vi "roboRIO v1.0 Reserve Encoder.vi"(7 "Allow multiple opens?":bool, 8 "error in (no error)":errorcluster, 10 "Encoder Channel":T2, 11 "myRIO FPGA Ref Out":T1) -> (0 "error out":errorcluster)   [LabVIEW 2021]
uses:
  <vilib>/myRIO/Common/Instrument Driver Framework/myRIO v1.0/Encoder/typedefs/Encoder Channels Enum.ctl
  <vilib>/myRIO/Common/Instrument Driver Framework/Utilities/typedefs/Generic FPGA Reference.ctl
  <vilib>/myRIO/Common/Instrument Driver Framework/roboRIO v1.0/Resource Manager/vis/roboRIO v1.0 Create Configuration List.vi
  <vilib>/myRIO/Common/Instrument Driver Framework/roboRIO v1.0/Resource Manager/vis/roboRIO v1.0 Reserve Channel.vi
  <vilib>/myRIO/Common/Instrument Driver Framework/roboRIO v1.0/Resource Manager/vis/roboRIO v1.0 Unreserve Channel.vi
  <vilib>/myRIO/Common/Instrument Driver Framework/roboRIO v1.0/Resource Manager/vis/roboRIO v1.0 Build Mutex Name.vi
  <vilib>/myRIO/Common/Instrument Driver Framework/Utilities/vis/IO Manager.vi
  <vilib>/Utility/error.llb/Error Cluster From Error Code.vi
  <vilib>/myRIO/Common/Instrument Driver Framework/Utilities/vis/Configuration Manager.vi
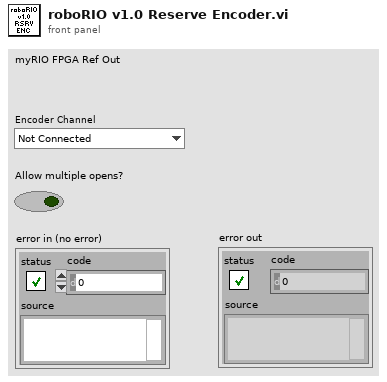
[diagram p1: front panel]
types:
  T1 = typedef "Generic FPGA Reference.ctl" = refnum<k20>
  T2 = typedef "Encoder Channels Enum.ctl" = enum16{"Not Connected", "C/ENC0", "C/ENC1", "A/ENC", "A/ENC0", "A/ENC1", "A/ENC2", "A/ENC3", "A/ENC4", "A/ENC5", "A/ENC6", "A/ENC7", "A/ENC8", "A/ENC9", "B/ENC", "B/ENC0", "B/ENC1", "B/ENC2", "B/ENC3", "B/ENC4", "B/ENC5", "B/ENC6", "B/ENC7", "B/ENC8", "B/ENC9", "DIO/ENC0", "DIO/ENC1", "DIO/ENC2", "DIO/ENC3", "DIO/ENC4"}
  T3 = typedef "roboRIO v1.0 Channel Reservation List.ctl" = T4[]
  T4 = typedef "roboRIO v1.0 Channel Reservation Info.ctl" = cluster{"Channel Name":string, "Connector":T5, "Mutex ID":i32}
  T5 = typedef "roboRIO v1.0 Connector List.ctl" = enum32{"None", "ConnectorB", "ConnectorI2C", "ConnectorDIO", "ConnectorRSL", "ConnectorRELAY", "ConnectorAI", "ConnectorPWM", "ConnectorSPI"}
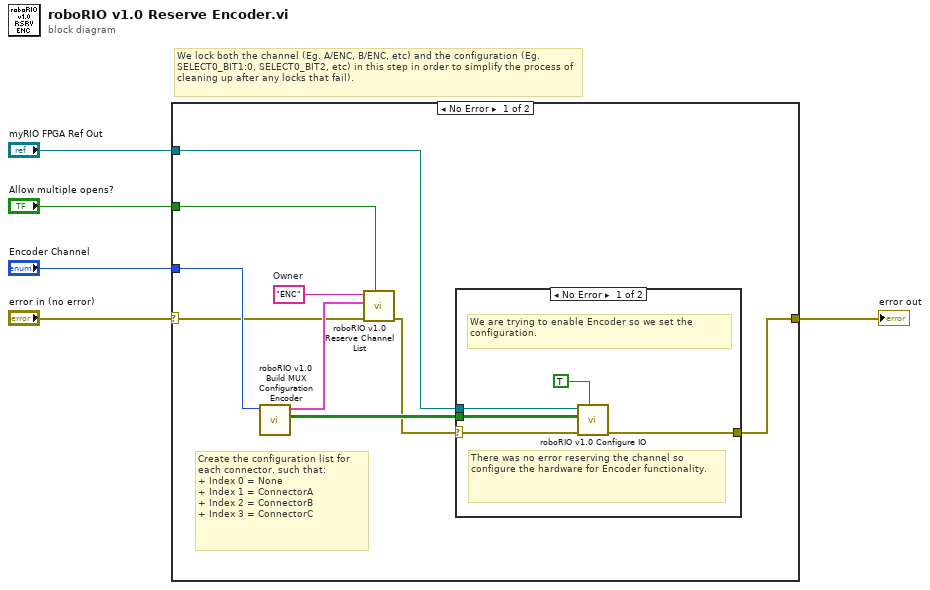
[diagram p0: block diagram]
diagram:
  # "We lock both the channel (Eg. A/ENC, B/ENC, etc) and the configuration (Eg. SELECT0_BIT1:0, SELECT0_BIT2, etc) in this step in order to simplify the process of cleaning up after any locks that fail)."
  n1 = case shown="No Error" "error in (no error)" {
    selector: "error in (no error)" -> [w9 w21]
    tunnel: "myRIO FPGA Ref Out" -> [w12 _]
    tunnel: "Encoder Channel" -> [w14 _]
    tunnel: [w6 w21] -> w3
    tunnel: "Allow multiple opens?" -> [w13 _]
    frame No Error {
      w10 = "ENC"  # Owner
      # "Create the configuration list for each connector. such that:\n+ Index 0 = None\n+ Index 1 = ConnectorA\n+ Index 2 = ConnectorB \n+ Index 3 = ConnectorC"
      n2 = call <vilib>:"roboRIO v1.0 Build MUX Configuration Encoder.vi"("Channel"=w14) -> ("Configuration Bitmask Array"=w8:bool[][], "Channel Reservation List"=w11:T3)  [unwired: 9 in]
      n3 = call <vilib>:"roboRIO v1.0 Reserve Channel List.vi"("Allow multiple opens?"=w13, "error in (no error)"=w9, "Channel Reservation List"=w11, "Owner"=w10) -> ("error out"=w7:errorcluster)  [unwired: 7 in]
      n4 = case shown="No Error" w7 {
        selector: w7 -> [w16 w20]
        tunnel: w12 -> [w19 _]
        tunnel: w8 -> [w17 _]
        tunnel: [w15 w20] -> w6
        frame No Error {
          # "There was no error reserving the channel so configure the hardware for Encoder functionality."
          # "We are trying to enable Encoder so we set the configuration."
          n5 = call <vilib>:"roboRIO v1.0 Configure IO.vi"("Value"=TRUE ("Clear?"), "error in (no error)"=w16, "Bitmask Array"=w17, "myRIO FPGA Ref In"=w19) -> ("error out"=w15:errorcluster)  [unwired: 7 in]
        }
        frame Error {
        }
      }
    }
    frame Error {
      # "Nothing to do since there is an incoming error."
    }
  }
  "error out" <- w3
